vi "Hella subvis check.vi"() -> ()   [LabVIEW 2013]
uses:
  CAN Communication/CAN Mode.ctl
panel:
  in  "CMD":u8
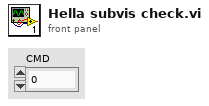
[diagram p1: front panel]
types:
  T1 = typedef "CAN Mode.ctl" = enum16{"Init", "Read", "Write", "Close"}
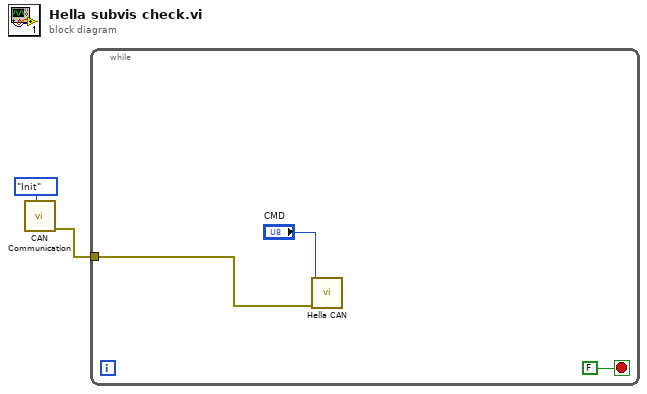
[diagram p0: block diagram]
diagram:
  n1 = call "CAN Communication.vi"("CAN Mode"=CAN_Mode."Init") -> ("Error OUT"=w1:errorcluster)  [unwired: 9 in, 1 out]
  n2 = while {
    tunnel: w1 -> [w3]
    stop <- FALSE stop-if-true
    n3 = call "Hella CAN.vi"("Error IN"=w3, "CMD"="CMD") -> ()  [unwired: 9 in, 1 out]
  }
